vi "Send Buffer Data to Reader.vi"(8 "error in (no error)":errorcluster, 9 "Buffer data":T1={"decimation"=0, "avg bandwidth"=0.0, "channels"=[], "byte order"=enum."big-endian", "buffer descriptor"={"buffer type"=enum."Engine", "plugin id"=0, "group id"=0, "transfer id"=0, "offset"=0, "length"=0}, "values channels"={"index"=0, "count"=0, "engine offset"=0}, "select start offset"=18446744073709551615, "select end offset"=0, "channel index"=-1} {"channels"."configuration"."string offset" format="%d bytes"; "avg bandwidth" format="%.0g bytes"}, 10 "server ID":refnum<k5>, 11 "queue":refnum<queue>) -> (0 "error out":errorcluster)   [LabVIEW 2017, in "Data Viewer.lvlib"]
uses:
  Core/VIs/Data Viewer/Source/Data Viewer.lvlib
  Buffer Reader/Queue Data.ctl
  Buffer Reader/Buffer Data.ctl
  Core/Classes/Configuration/Core/Transfer/Channel Configuration.ctl
  Core/Typedefs/Core Channel Configuration.ctl
  Core/Typedefs/DSF Data Type.ctl
  Core/Typedefs/DSF Settings Info.ctl
  Core/Typedefs/DSF Byte Order.ctl
  Core/Classes/Thread/Data Server/DSF Buffer Subset Descriptor.ctl
  Core/Typedefs/DSF Buffer Type.ctl
  Values Channels.ctl
  Core/DSF Core.lvlib
  Core/Classes/Configuration/Core/Channel/Channel Configuration.lvclass
  Core/Classes/Configuration/Core/Transfer/Transfer Configuration.lvclass
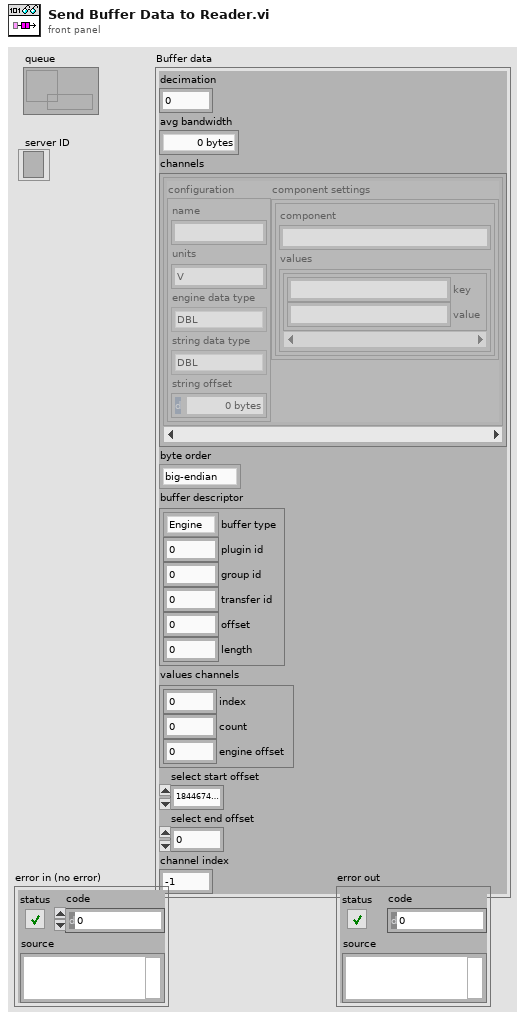
[diagram p1: front panel]
types:
  T1 = typedef "Data Viewer.lvlib/Buffer Data.ctl" = cluster{"decimation":u64, "avg bandwidth":dbl, "channels":T2[], "byte order":T6, "buffer descriptor":T7, "values channels":T9, "select start offset":u64, "select end offset":u64, "channel index":i32}
  T2 = typedef "DSF Core.lvlib/Transfer Configuration.lvclass/Channel Configuration.ctl" = cluster{"configuration":T3, "component settings":T5[]}
  T3 = typedef "DSF Core.lvlib/Channel Configuration.lvclass/Core Channel Configuration.ctl" = cluster{"name":string, "units":string, "engine data type":T4, "string data type":T4, "string offset":u64}
  T4 = typedef "DSF Core.lvlib/DSF Data Type.ctl" = enum8{"Bool", "SGL", "DBL", "I8", "I16", "I32", "I64", "U8", "U16", "U32", "U64"}
  T5 = typedef "DSF Core.lvlib/DSF Settings Info.ctl" = cluster{"component":string, "values":cluster{"key":string, "value":string}[]}
  T6 = typedef "DSF Core.lvlib/DSF Byte Order.ctl" = enum8{"big-endian", "little-endian"}
  T7 = typedef "DSF Core.lvlib/DSF Buffer Subset Descriptor.ctl" = cluster{"buffer type":T8, "plugin id":i32, "group id":i32, "transfer id":i32, "offset":u64, "length":i64}
  T8 = typedef "DSF Core.lvlib/DSF Buffer Type.ctl" = enum16{"Engine", "String"}
  T9 = typedef "Data Viewer.lvlib/Values Channels.ctl" = cluster{"index":i32, "count":i32, "engine offset":u64}
  T10 = typedef "Data Viewer.lvlib/Queue Data.ctl" = cluster{"server ID":refnum<k5>, "Buffer data":T1}
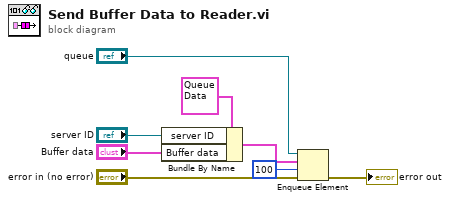
[diagram p0: block diagram]
diagram:
  n1 = Bundle By Name(cluster=T10 {"server ID"=refnum, "Buffer data"={"decimation"=0, "avg bandwidth"=0.0, "channels"=[], "byte order"=enum."little-endian", "buffer descriptor"={"buffer type"=enum."Engine", "plugin id"=0, "group id"=0, "transfer id"=0, "offset"=0, "length"=0}, "values channels"={"index"=0, "count"=0, "engine offset"=0}, "select start offset"=18446744073709551615, "select end offset"=0, "channel index"=-1}} ("element"), "server ID"="server ID", "Buffer data"="Buffer data") -> (w5:T10)
  n2 = Enqueue Element(queue="queue", element=w5, timeout in ms (-1)=100, error in (no error)="error in (no error)") -> (error out=→"error out":errorcluster)  [unwired: 2 out]
